vi "uTTA_GenerateErrorClusters.vi"() -> ()   [LabVIEW 2021]
uses:
  <vilib>/Utility/error.llb/DialogType.ctl
  3d39b208-b984-4a20-8744-b1eefe72efce.vi
  <vilib>/Comparison/Less/Less Functor/Less Functor.lvclass
panel:
  out "Type of Dialog":T1[](array[typedef]) items=["no dialog", "OK message", "continue or stop message", "OK message + warnings", "continue/stop + warnings"]
  out "Error Messages":string[](array[string])
  out "Error Codes":i32[](array[numeric])
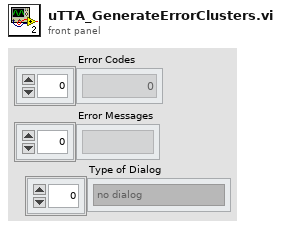
[diagram p1: front panel]
types:
  T1 = typedef "DialogType.ctl" = u16
  T2 = cluster{"Error Code":i32, "Message":string, "type of dialog":T1}[]
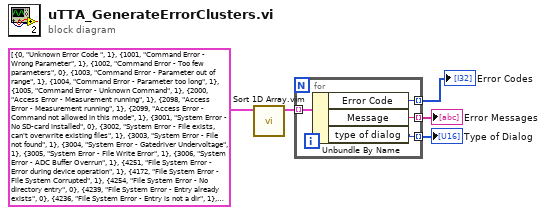
[diagram p0: block diagram]
diagram:
  n1 = call "Sort 1D Array.vim"("unsorted array"=T2 [{"Error Code"=0, "Message"="Unknown Error Code ", "type of dialog"=1}, {"Error Code"=1001, "Message"="Command Error - Wrong Parameter", "type of dialog"=1}, {"Error Code"=1002, "Message"="Command Error - Too few parameters", "type of dialog"=0}, {"Error Code"=1003, "Message"="Command Error - Parameter out of range", "type of dialog"=1}, {"Error Code"=1004, "Message"="Command Error - Parameter too long", "type of dialog"=1}, {"Error Code"=1005, "Message"="Command Error - Unknown Command", "type of dialog"=1}, {"Error Code"=2000, "Message"="Access Error - Measurement running", "type of dialog"=1}, {"Error Code"=2098, "Message"="Access Error - Measurement running", "type of dialog"=1}, {"Error Code"=2099, "Message"="Access Error - Command not allowed in this mode", "type of dialog"=1}, {"Error Code"=3001, "Message"="System Error - No SD-card installed", "type of dialog"=0}, {"Error Code"=3002, "Message"="System Error - File exists, can't overwrite existing files", "type of dialog"=1}, {"Error Code"=3003, "Message"="System Error - File not found", "type of dialog"=1}, {"Error Code"=3004, "Message"="System Error - Gatedriver Undervoltage", "type of dialog"=1}, {"Error Code"=3005, "Message"="System Error - File Write Error", "type of dialog"=1}, {"Error Code"=3006, "Message"="System Error - ADC Buffer Overrun", "type of dialog"=1}, {"Error Code"=4251, "Message"="File System Error - Error during device operation", "type of dialog"=1}, {"Error Code"=4172, "Message"="File System Error - File System Corrupted", "type of dialog"=1}, {"Error Code"=4254, "Message"="File System Error - No directory entry", "type of dialog"=0}, {"Error Code"=4239, "Message"="File System Error - Entry already exists", "type of dialog"=0}, {"Error Code"=4236, "Message"="File System Error - Entry is not a dir", "type of dialog"=1}, {"Error Code"=4235, "Message"="File System Error - Entry is a dir", "type of dialog"=1}, {"Error Code"=4217, "Message"="File System Error - Dir is not empty", "type of dialog"=0}, {"Error Code"=4247, "Message"="File System Error - Bad file number", "type of dialog"=0}, {"Error Code"=4229, "Message"="File System Error - File too large", "type of dialog"=3}, {"Error Code"=4234, "Message"="File System Error - Invalid parameter", "type of dialog"=1}, {"Error Code"=4228, "Message"="File System Error - No space left on device", "type of dialog"=1}, {"Error Code"=4244, "Message"="File System Error - No more memory available", "type of dialog"=1}, {"Error Code"=4195, "Message"="File System Error - No data/attr available", "type of dialog"=1}, {"Error Code"=4220, "Message"="File System Error - File name too long", "type of dialog"=0}]) -> ("sorted array"=w4:T2)  [unwired: 10 in]
  n2 = for {
    tunnel: w4 -> [w9] mode=indexing
    tunnel: [w8] -> w3 mode=indexing
    tunnel: [w7] -> w2 mode=indexing
    tunnel: [w6] -> w1 mode=indexing
    n3 = Unbundle By Name(w9) -> ("Error Code"=w8:i32, "Message"=w7:string, "type of dialog"=w6:T1)
  }
  "Error Codes" <- w3
  "Error Messages" <- w2
  "Type of Dialog" <- w1
